vi "TCP Send Command.vi"(8 "error in":errorcluster, 11 "Command":string) -> (0 "error out":errorcluster, 3 "connection ID out":refnum<k5>)   [LabVIEW 2013]
doc: "This VI implements a client for the TCP Named Service - Server.vi. It connects to a service by specifying the server address and the name of the service. The client receives the string sent by the server, displays the string and closes the connection."
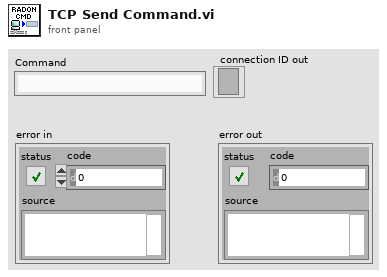
[diagram p1: front panel]
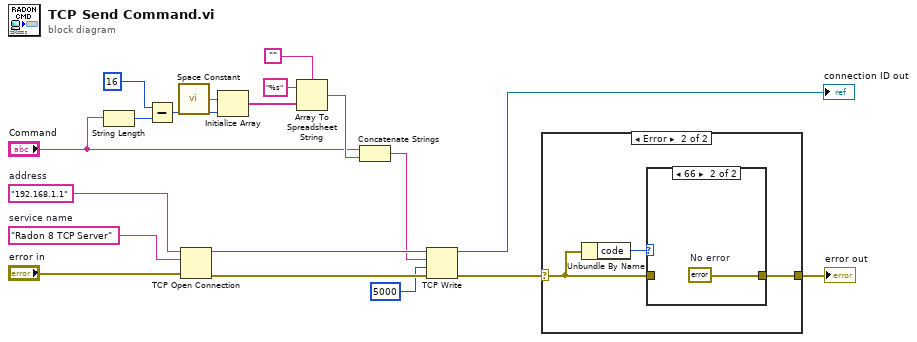
[diagram p0: block diagram]
diagram:
  w18 = "Radon 8 TCP Server"  # service name
  w19 = "192.168.1.1"  # address
  n1 = String Length(string="Command") -> (length=w13:i32)
  n2 = Subtract(x=16 ("length"), y=w13) -> (x-y=w11:i32)
  n3 = call <vilib>:"Space Constant.vi"() -> ("String"=w10:string)
  n4 = TCP Open Connection(address=w19, remote port or service name=w18, error in (no error)="error in") -> (connection ID=w17:refnum<k5>, error out=w16:errorcluster)  [unwired: 2 in]
  n5 = Initialize Array(w10, w11) -> (w9:string[])
  n6 = Array To Spreadsheet String(delimiter (Tab)="", array=w9, 3:"%s" ("format string")) -> (spreadsheet string=w6:string)
  n7 = Concatenate Strings("Command", w6) -> (w4:string)
  n8 = TCP Write(connection ID=w17, data in=w4, error in (no error)=w16, 9:5000 ("timeout ms (25000)")) -> (connection ID out=→"connection ID out":refnum<k5>, error out=w3:errorcluster)  [unwired: 1 out]
  n9 = case shown="Error" w3 {
    selector: w3 -> [w20 w22]
    tunnel: [w20 w21] -> w14
    frame No Error {
    }
    frame Error {
      n10 = Unbundle By Name(w22) -> ("code"=w23:i32)
      n11 = case shown="66" w23 {
        tunnel: w22 -> [w24 _]
        tunnel: [w24 w25] -> w21
        frame Default {
        }
        frame 66 {
          w25 = errorcluster {"status"=FALSE, "code"=0, "source"=""}  # No error
        }
      }
    }
  }
  "error out" <- w14
